vi "SetParameters (SubVI).vi"(0 "Stop":refnum<vi>, 1 "Pannel User Message":refnum<vi>, 3 "DAQmx Device Name":tag, 5 "VISA resource name in":refnum<visa-resource-name>, 7 "PN":string, 9 "Motor Speed RPM Serial":refnum<vi>, 11 "error in (no error)":errorcluster, 12 "FileName":string) -> (15 "error out":errorcluster)   [LabVIEW 2017]
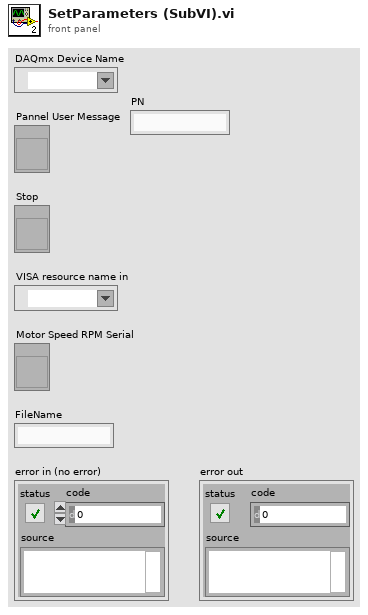
[diagram p1: front panel]
types:
  T1 = enum16{"Init", "0 ohm", "6 ohm", "13.2 ohm", "15 ohm", "25.9 ohm", "33 ohm", "Down", "Up", "Venable", "Firmware", "PowerSuply"}[]
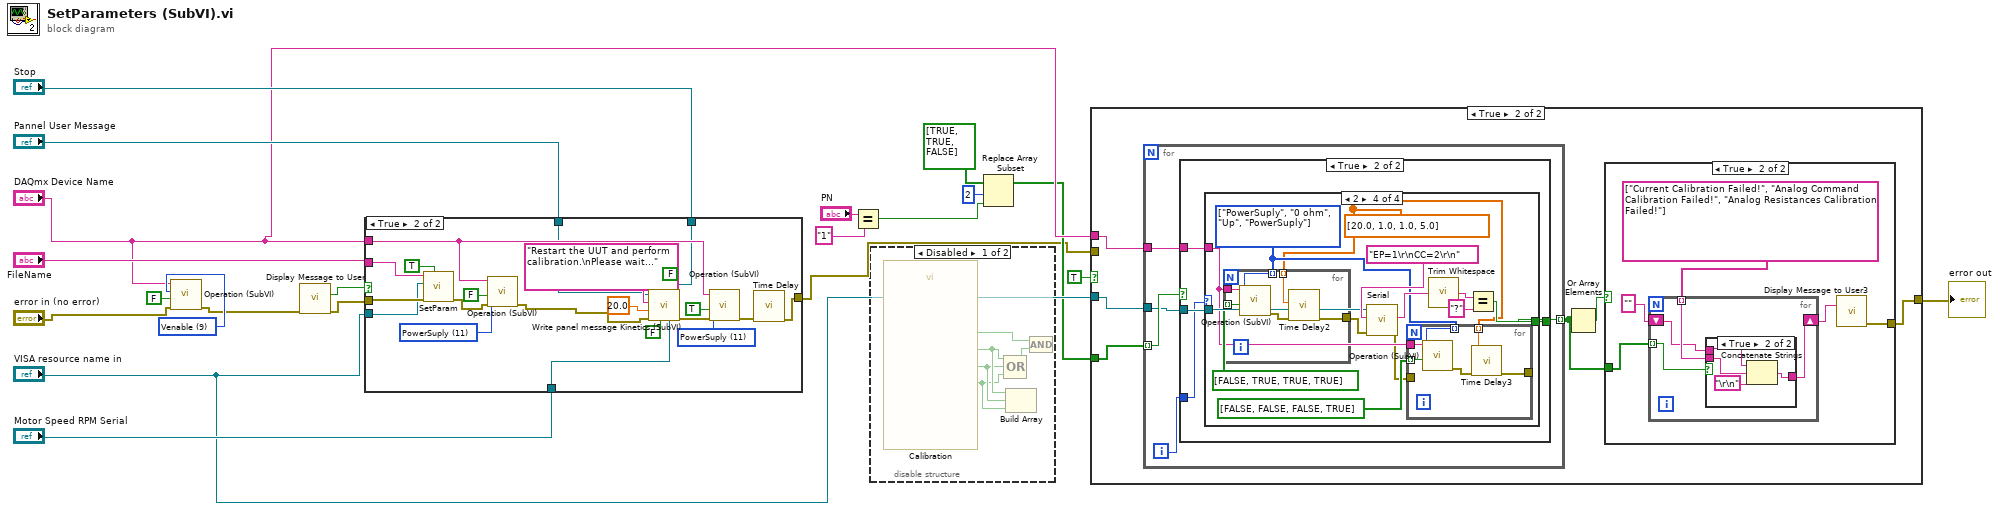
[diagram p0: block diagram]
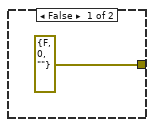
[diagram p4: hidden frame]
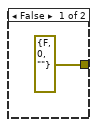
[diagram p5: hidden frame]
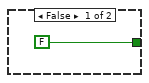
[diagram p7: hidden frame]
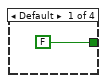
[diagram p8: hidden frame]
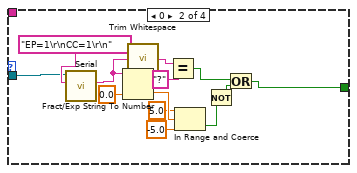
[diagram p9: hidden frame]
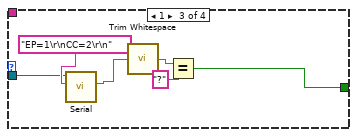
[diagram p10: hidden frame]
diagram:
  w16 = u16 9 items=["Init", "0 ohm", "6 ohm", "13.2 ohm", "15 ohm", "25.9 ohm", "33 ohm", "Down", "Up", "Venable", "Firmware", "PowerSuply"] ("Operation")
  n1 = call "Operation (SubVI).vi"("error in (no error)"="error in (no error)", "On/Off"=FALSE, "Operation"=w16, "DAQmx Device Name"="DAQmx Device Name") -> ("error out"=w13:errorcluster)  [unwired: 7 in]
  n2 = call "Display Message to User"("error in (no error)"=w13) -> ("error out"=w9:errorcluster, "Yes"=w10:bool)  [unwired: 9 in]
  n3 = case shown="True" w10 {
    tunnel: w9 -> [w22 w43]
    tunnel: [w22 w29] -> w1
    tunnel: "VISA resource name in" -> [_ w24]
    tunnel: "FileName" -> [_ w38]
    tunnel: "DAQmx Device Name" -> [_ w28]
    tunnel: "Pannel User Message" -> [_ w27]
    tunnel: "Stop" -> [_ w26]
    tunnel: "Motor Speed RPM Serial" -> [_ w25]
    frame False {
    }
    frame True {
      w32 = u16 11 items=["Init", "0 ohm", "6 ohm", "13.2 ohm", "15 ohm", "25.9 ohm", "33 ohm", "Down", "Up", "Venable", "Firmware", "PowerSuply"] ("Operation")
      w36 = u16 11 items=["Init", "0 ohm", "6 ohm", "13.2 ohm", "15 ohm", "25.9 ohm", "33 ohm", "Down", "Up", "Venable", "Firmware", "PowerSuply"] ("Operation")
      n4 = call "SetParam.vi"("RS"=TRUE, "error in (no error)"=w43, "Visa"=w24, "Filein"=w38) -> ("error out"=w34:errorcluster)  [unwired: 7 in]
      n5 = call "Operation (SubVI).vi"("error in (no error)"=w34, "On/Off"=FALSE, "Operation"=w36, "DAQmx Device Name"=w28) -> ("error out"=w23:errorcluster)  [unwired: 7 in]
      n6 = call "Write panel message Kinetics (SubVI).vi"(4:"rpm"=w25, 5:"rpm"=FALSE ("rpm"), "PrintTime"=FALSE, "Stop"=w26, "error in (no error)"=w23, "Time to wait"=20.0, "Strin"="Restart the UUT and perform calibration.\nPlease wait...", "String in"=w27) -> ("error out"=w31:errorcluster)  [unwired: 2 in, 1 out]
      n7 = call "Operation (SubVI).vi"("error in (no error)"=w31, "On/Off"=TRUE, "Operation"=w32, "DAQmx Device Name"=w28) -> ("error out"=w30:errorcluster)  [unwired: 7 in]
      n8 = call "Time Delay"("error in (no error)"=w30) -> ("error out"=w29:errorcluster)  [unwired: 10 in]
    }
  }
  n9 = Equal?(x="PN", y="1") -> (x = y?=w4:bool)
  n10 = disable-structure shown="Disabled" {
    frame Disabled {
      n11 = call "Calibration"() -> ("Analog Resistances"=w44:bool, "Analog Command"=w45:bool, "Current"=w46:bool, "OK"=w48:bool)  [unwired: 15 in, 1 out]
      n12 = Compound Arithmetic op=OR(w46, w45, w44) -> (w47:bool)
      n13 = Build Array(w46, w45, w44) -> ()  [unwired: 1 out]
      n14 = Compound Arithmetic op=AND(w48, w47) -> ()  [unwired: 1 out]
    }
    frame Enabled {
    }
  }
  n15 = Replace Array Subset(array=bool[] [TRUE, TRUE, FALSE], new element=w4, index=2) -> (w2:bool[])
  n16 = case shown="True" TRUE {
    tunnel: w2 -> [_ w55]
    tunnel: "DAQmx Device Name" -> [_ w53]
    tunnel: "VISA resource name in" -> [_ w54]
    tunnel: [errorcluster {"status"=FALSE, "code"=0, "source"=""} ("error out") w50] -> w11
    tunnel: w1 -> [_ _]
    frame False {
    }
    frame True {
      n17 = for {
        tunnel: w55 -> [w75] mode=indexing
        tunnel: w54 -> [w74]
        tunnel: [w73] -> w51 mode=indexing
        tunnel: w53 -> [w71]
        i -> [w72]
        n18 = case shown="True" w75 {
          tunnel: w74 -> [_ w80]
          tunnel: [FALSE w79] -> w73
          tunnel: w72 -> [_ w78]
          tunnel: w71 -> [_ w77]
          frame False {
          }
          frame True {
            n19 = case shown="2" w78 {
              tunnel: w80 -> [_ w93 w99 w112]
              tunnel: [FALSE w82 w96 w109] -> w79
              tunnel: w77 -> [_ _ _ w102]
              frame Default {
              }
              frame 0 {
                n20 = call "Serial.vi"("write buffer"="EP=1\r\nCC=1\r\n", "VISA resource name"=w93) -> ("read buffer"=w85:string)  [unwired: 8 in, 1 out]
                n21 = Fract/Exp String To Number(string=w85, default (0 dbl)=0.0 ("default (0 DBL)")) -> (number=w91:dbl)  [unwired: 2 in, 1 out]
                n22 = call <vilib>:"Trim Whitespace.vi"("string"=w85) -> ("trimmed string"=w87:string)  [unwired: 1 in]
                n23 = Equal?(x=w87, y="?") -> (x = y?=w86:bool)
                n24 = In Range and Coerce(upper limit=5.0, x=w91, lower limit=-5.0) -> (In Range?=w84:bool)  [unwired: 1 out]
                n25 = Not(x=w84) -> (.not. x?=w83:bool)
                n26 = Or(x=w86, y=w83) -> (x .or. y?=w82:bool)
              }
              frame 1 {
                n27 = call "Serial.vi"("write buffer"="EP=1\r\nCC=2\r\n", "VISA resource name"=w99) -> ("read buffer"=w95:string)  [unwired: 8 in, 1 out]
                n28 = call <vilib>:"Trim Whitespace.vi"("string"=w95) -> ("trimmed string"=w97:string)  [unwired: 1 in]
                n29 = Equal?(x=w97, y="?") -> (x = y?=w96:bool)
              }
              frame 2 {
                w104 = dbl[] [20.0, 1.0, 1.0, 5.0]
                w105 = T1 [enum."PowerSuply", enum."0 ohm", enum."Up", enum."PowerSuply"] items=["Init", "0 ohm", "6 ohm", "13.2 ohm", "15 ohm", "25.9 ohm", "33 ohm", "Down", "Up", "Venable", "Firmware", "PowerSuply"]
                n30 = for {
                  tunnel: w102 -> [w125]
                  tunnel: bool[] [FALSE, TRUE, TRUE, TRUE] -> [w124] mode=indexing
                  tunnel: w105 -> [w123] mode=indexing
                  tunnel: [w121] -> w106
                  tunnel: w104 -> [w120] mode=indexing
                  n31 = call "Operation (SubVI).vi"("On/Off"=w124, "Operation"=w123, "DAQmx Device Name"=w125) -> ("error out"=w122:errorcluster)  [unwired: 8 in]
                  n32 = call "Time Delay2"("error in (no error)"=w122, "Delay Time (s)"=w120) -> ("error out"=w121:errorcluster)  [unwired: 9 in]
                }
                n33 = call "Serial.vi"("error in (no error)"=w106, "write buffer"="EP=1\r\nCC=2\r\n", "VISA resource name"=w112) -> ("error out"=w101:errorcluster, "read buffer"=w108:string)  [unwired: 7 in]
                n34 = for {
                  tunnel: w102 -> [w119]
                  tunnel: bool[] [FALSE, FALSE, FALSE, TRUE] -> [w118] mode=indexing
                  tunnel: w105 -> [w117] mode=indexing
                  tunnel: [w115] -> _
                  tunnel: w104 -> [w114] mode=indexing
                  tunnel: w101 -> [_]
                  n35 = call "Operation (SubVI).vi"("On/Off"=w118, "Operation"=w117, "DAQmx Device Name"=w119) -> ("error out"=w116:errorcluster)  [unwired: 8 in]
                  n36 = call "Time Delay3"("error in (no error)"=w116, "Delay Time (s)"=w114) -> ("error out"=w115:errorcluster)  [unwired: 9 in]
                }
                n37 = call <vilib>:"Trim Whitespace.vi"("string"=w108) -> ("trimmed string"=w110:string)  [unwired: 1 in]
                n38 = Equal?(x=w110, y="?") -> (x = y?=w109:bool)
              }
            }
          }
        }
      }
      n39 = Or Array Elements(Boolean array=w51) -> (logical OR=w52:bool)
      n40 = case shown="True" w52 {
        tunnel: [errorcluster {"status"=FALSE, "code"=0, "source"=""} ("error out") w58] -> w50
        tunnel: w51 -> [_ w57]
        frame False {
        }
        frame True {
          n41 = for {
            tunnel: w57 -> [w65] mode=indexing
            shift-right: [w63] -> w61
            shift-left: "" -> [w62]
            tunnel: string[] ["Current Calibration Failed!", "Analog Command Calibration Failed!", "Analog Resistances Calibration Failed!"] -> [w64] mode=indexing
            n42 = case shown="True" w65 {
              tunnel: w64 -> [_ w69]
              tunnel: [w66 w68] -> w63
              tunnel: w62 -> [w66 w67]
              frame False {
              }
              frame True {
                n43 = Concatenate Strings(w67, w69, "\r\n") -> (w68:string)
              }
            }
          }
          n44 = call "Display Message to User3"("Message"=w61) -> ("error out"=w58:errorcluster)  [unwired: 9 in, 1 out]
        }
      }
    }
  }
  "error out" <- w11
